vi "Show Error Details.vi"(8 "error in (no error)":errorcluster, 10 "Error Info":T1 {"Time Stamp" format="%<%x %.3X>T"}, 11 "Error Manager in":refnum<class "Error Manager.lvclass">) -> (0 "error out":errorcluster, 3 "Error Manager out":refnum<class "Error Manager.lvclass">)   [LabVIEW 2026, in "TALOS.lvlib" / "Error Manager.lvlib" / "Error Manager.lvclass"]
uses:
  Error Manager.lvclass
  C:/LabVIEW Code/TALOS/talos/Father of all uServices/Father of all uServices/Father of all uServices.lvclass
  Error Info.ctl
  Ancestor/Ancestor/Ancestor.lvclass/Ancestor.ctl
  Support VIs/Generate Error.vi
  FGV/Error Memory/Get Error Description.vi
  Support VIs/Get PC name.vi
  Ancestor/Ancestor/Read ID.vi
  Support VIs/Get Class Name.vi
  <vilib>/Utility/error.llb/Clear Errors.vi
  FGV/Error Memory/Error Memory Core.vi
  <vilib>/AdvancedString/Delimited String to 1D String Array.vi
  <vilib>/AdvancedString/Delimited String to 1D String Array (string).vi
  Support VIs/Circus Root Path.vi
  FGV/Error Memory/Error Crt Lvl checker.vi
  FGV/Error Memory/Error Memory Core.vi/40c8088d-b597-4017-91af-faa98e00292e.vi
  FGV/Error Memory/Error Memory Core.vi/d4a3ab98-063c-4e44-b43d-fbdcfe6c2be2.vi
  Support VIs/Global Memory.vi
  <vilib>/Utility/LVClass/Get LV Class Name.vi
  Support VIs/Is in Packed Library.vi
  Support VIs/TALOS Root path.vi
  Support VIs/Read CSV worksheet.vi
  Support VIs/Global Constants.vi
  <vilib>/Utility/error.llb/General Error Handler.vi
  Support VIs/Error Log.vi
  Ancestor/Ancestor/Ancestor.lvclass
  <vilib>/Comparison/Equal/Equal Functor/Equal Functor.lvclass
  Father of all uServices/Father of all uServices/Father of all uServices.lvclass
  <vilib>/MultiError/TokenizeJSON/Multi Error Cluster.lvlib
  TALOS.lvlib
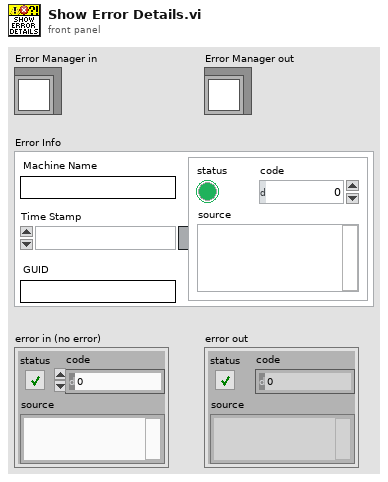
[diagram p1: front panel]
types:
  T1 = typedef "TALOS.lvlib/Error Manager.lvlib/Error Manager.lvclass/Error Info.ctl" = cluster{"error out":errorcluster, "Time Stamp":timestamp, "Machine Name":string, "GUID":string}
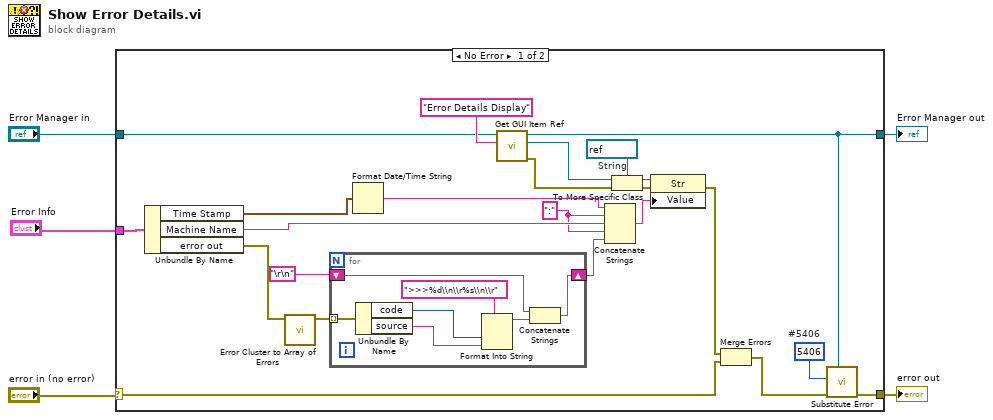
[diagram p0: block diagram]
diagram:
  n1 = case shown="No Error" "error in (no error)" {
    selector: "error in (no error)" -> [w13 w36]
    tunnel: [w9 w37] -> w4
    tunnel: "Error Manager in" -> [w25 w37]
    tunnel: "Error Info" -> [w24 _]
    tunnel: [w11 w36] -> w1
    frame No Error {
      w6 = ":" ("string")
      w12 = 5406  # #5406
      w28 = refnum<vi> refnum  # String
      n2 = Unbundle By Name(w24) -> ("Time Stamp"=w20:timestamp, "Machine Name"=w19:string, "error out"=w23:errorcluster)
      n3 = call <vilib>:"Error Cluster to Array of Errors.vi"("error"=w23) -> ("array of errors"=w21:errorcluster[])  [unwired: 10 in]
      n4 = for {
        tunnel: w21 -> [w35] mode=indexing
        shift-right: [w31] -> w7
        shift-left: "\r\n" -> [w29]
        n5 = Unbundle By Name(w35) -> ("code"=w34:i32, "source"=w33:string)
        n6 = Format Into String(format string=">>>%d\\n\\r%s\\n\\r", w34, w33) -> (resulting string=w30:string)  [unwired: 2 in, 1 out]
        n7 = Concatenate Strings(w29, w30) -> (w31:string)
      }
      n8 = Format Date/Time String(seconds (now)=w20) -> (date/time string=w8:string)  [unwired: 2 in]
      n9 = call "Get GUI Item Ref.vi"("FP Item Name"="Error Details Display", "uService Template in"=w25) -> ("error out"=w16:errorcluster, "Ctl Refnum"=w27:refnum<vi>, "uService Template out"=w9:refnum<class "Error Manager.lvclass">)  [unwired: 7 in]
      n10 = Concatenate Strings(w8, w6, w19, w6, w7) -> (w17:string)
      n11 = To More Specific Class(target class=w28, reference=w27, error in=w16) -> (specific class reference=w22:refnum<vi>, error out=w15:errorcluster)
      n12 = property class="Str"(reference=w22, error in=w15, "Value"=w17) -> (error out=w14:errorcluster)  [unwired: 1 out]
      n13 = Merge Errors(w14, w13) -> (w10:errorcluster)
      n14 = call "Substitute Error.vi"("LabVIEW Object"=w9, "error in (no error)"=w10, "Error Code"=w12) -> ("error out"=w11:errorcluster)  [unwired: 8 in]
    }
    frame Error {
    }
  }
  "error out" <- w1
  "Error Manager out" <- w4
